vi "HFRR ADV v01.vi"() -> ()   [LabVIEW 2025] (continued)
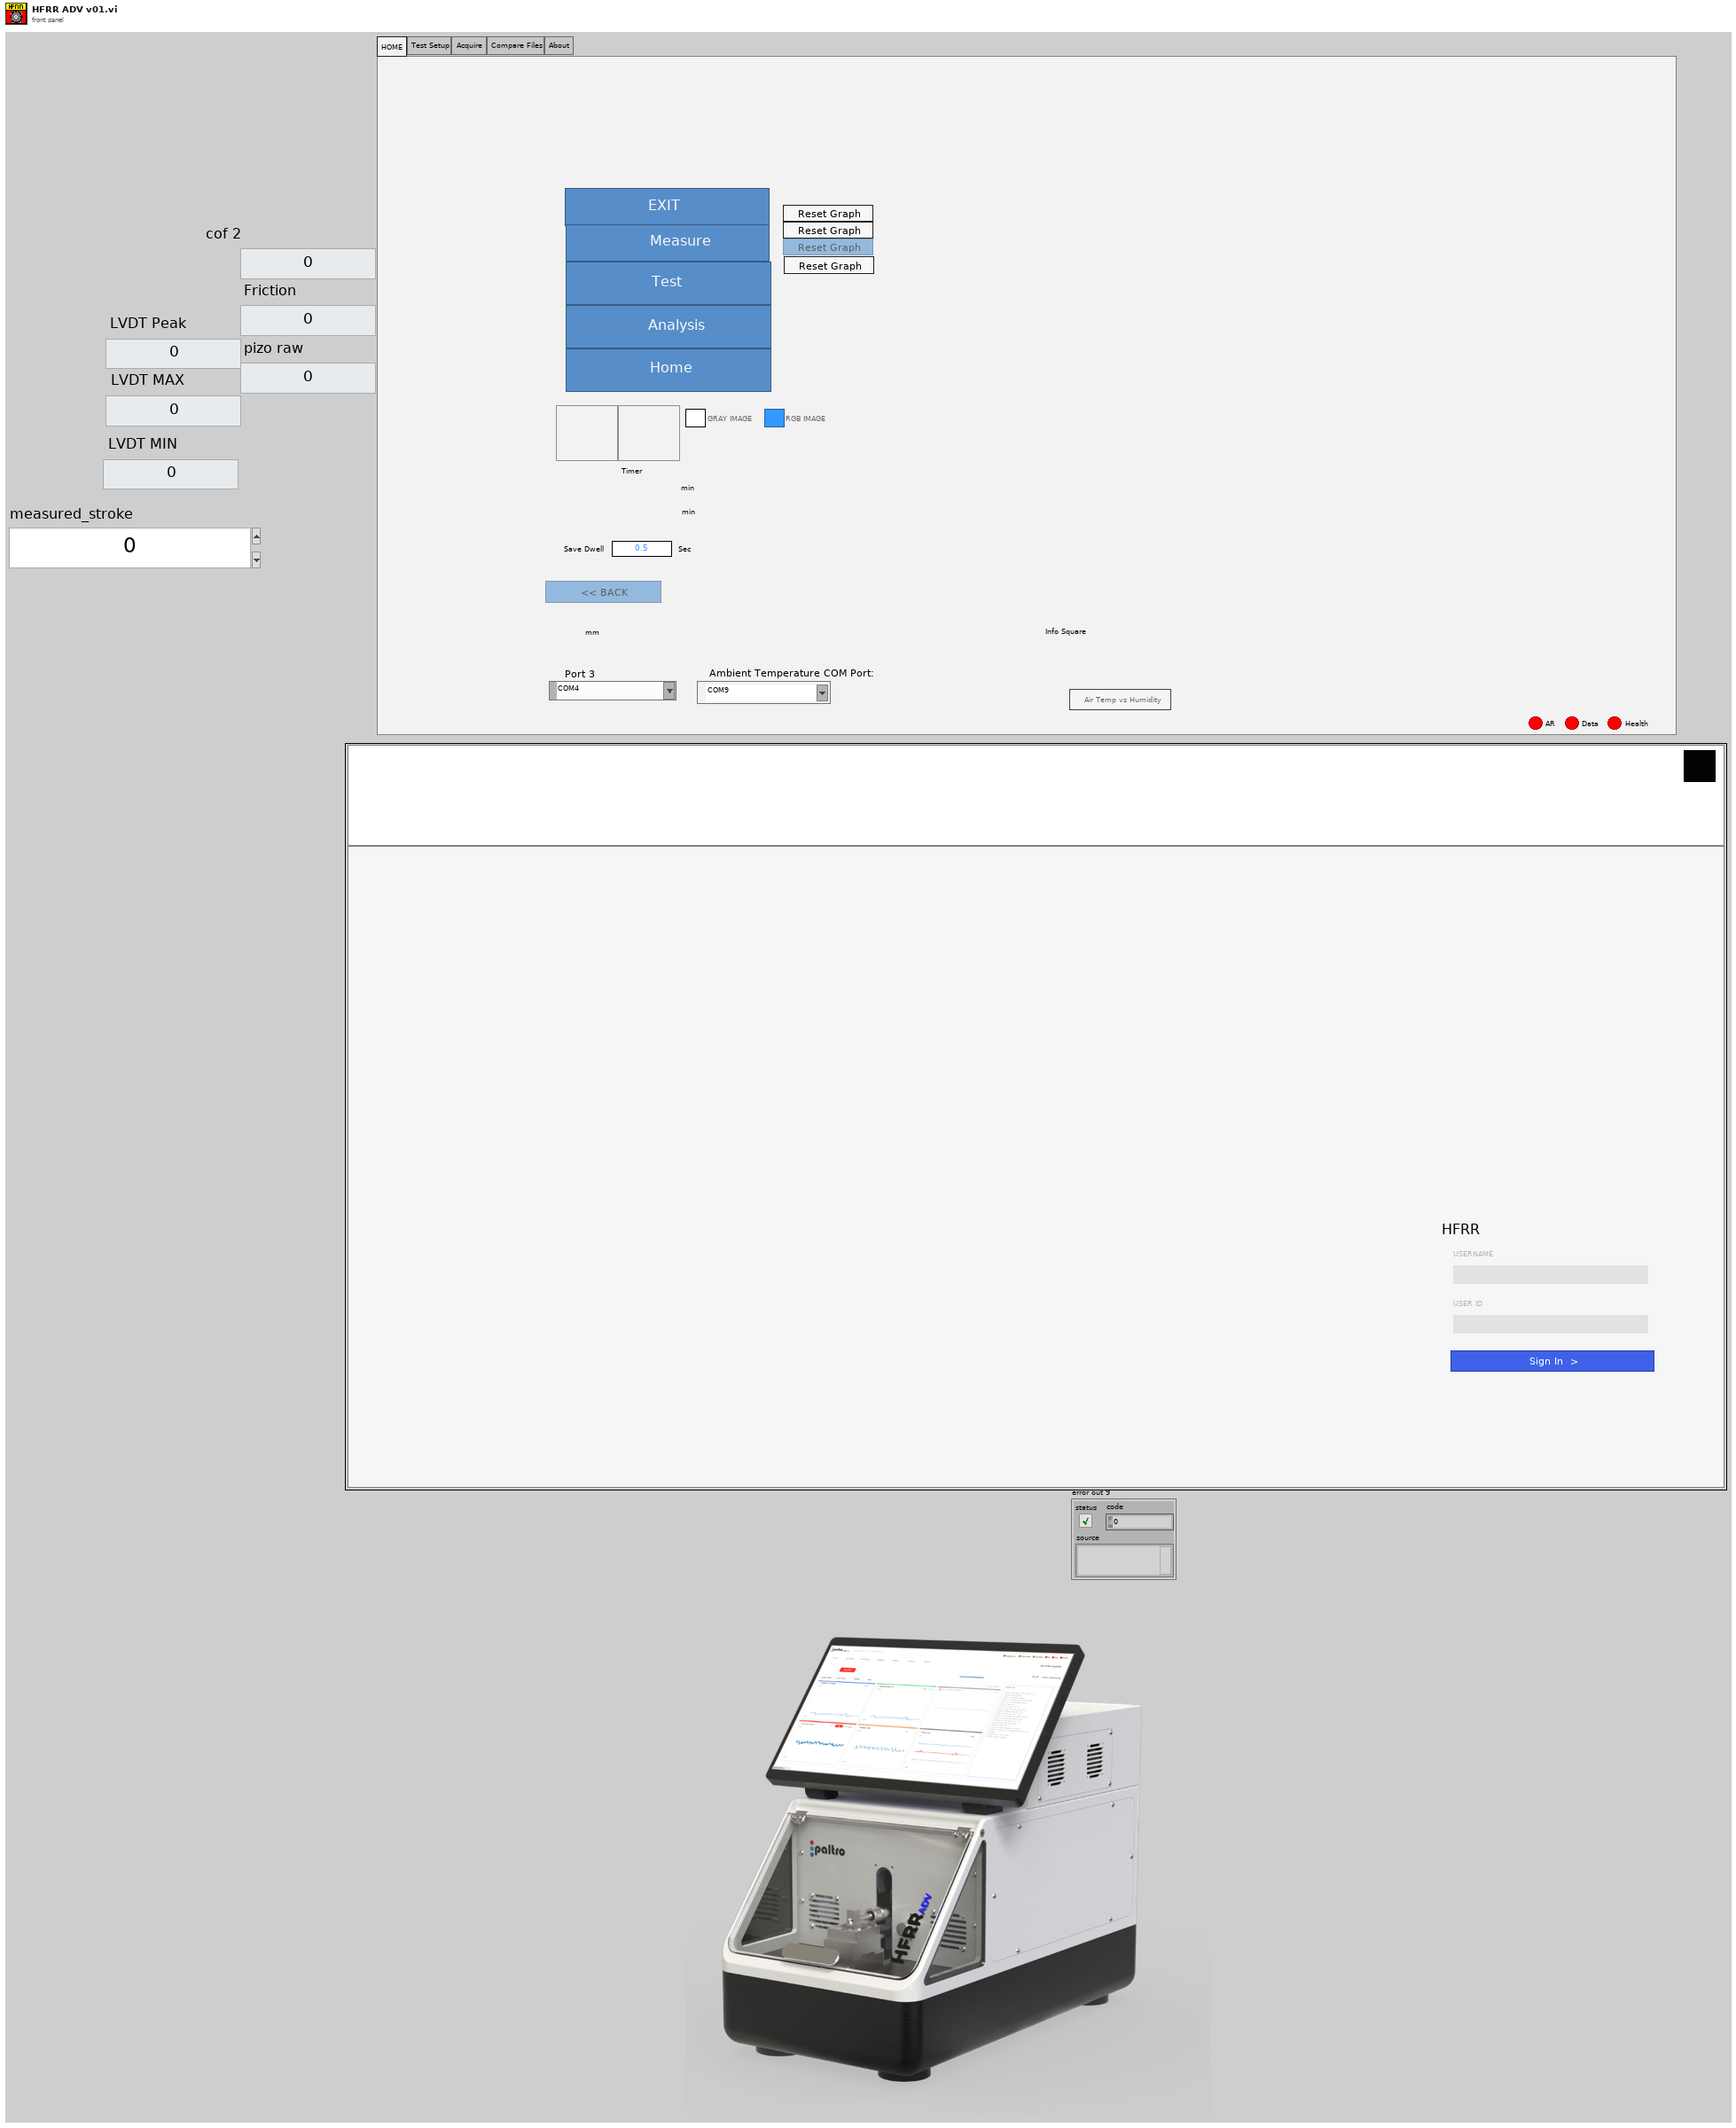
[diagram p1: front panel]
types:
  T1 = enum32{"Home", "Dashboard", "Imaging", "Report", "Analysis", "About", "Test Setup", "Advance"}
  T2 = enum32{"HOME", "Test Setup", "Acquire", "Adv Scar", "Adv Scar Report", "Compare Files", "About", "Advance", "Mooha"}
  T3 = enum16{"ASTM D6079", "ISO 12156", "CEC F-096-A-06", "Custom"}
  T4 = enum32{"Dashboard 1", "Dashboard 2", "Dashboard 3"}
  T5 = enum32{"COF", "Friction", "ECR", "Temperature", "Humidity", "Stroke"}
  T6 = enum32{"Coefficient Of Friction", "Air Temperature", "Humidity", "Stroke", "Sample Temperature", "Electrical Contact Resistance", "Frequency", "Air Temp vs Rh"}
  T7 = enum32{"Gains", "Configuration Parameters", "Temperature Calibration"}
  T8 = enum32{"Stroke Data", "Temperature Calibration", "Friction Force Raw Data"}
  T9 = enum32{"Temp Variables", "Camera", "WO 2465 (1)", "WO 2465 (2)", "WO 2465 (3)"}
  T10 = typedef "Auto Start enum.ctl" = enum16{"Init", "Humidity & Temperature On", "Reach point", "Maintain Stage", "Start Stage", "close", "Exit"}
  T11 = enum32{"Freqz control", "Low Speed Analog Inputs & Digital IOs", "Temperature Tuning", "Voltage LVDT raw", "High Speed Analog Inputs - Displacement & Friction", "LVDT Calibration", "Sericve", "Friction Force Calibration", "Bytes At Port", "Loadcell Board"}
  T12 = cluster{"proportional gain (Kc)":dbl, "integral time (Ti, min)":dbl, "derivative time (Td, min)":dbl}
  T13 = typedef "imagedata.ctl" = cluster{"image type":i32, "image depth":i32, "image":u8[], "mask":u8[], "colors":u32[], "Rectangle":cluster{"left":i16, "top":i16, "right":i16, "bottom":i16}}
  T14 = enum32{"HOME", "Test Setup", "Acquire", "Compare Files", "Print Report", "About", "Advance", "Mooha"}
  T15 = enum8{"Enabled", "Disabled", "Disabled and Grayed Out"}
  T16 = cluster{"Read Heave and Surge":string, "Bytes at Heave Port":dbl, "Heave and Surge COM Port:":refnum<visa-resource-name>, "Com Port 2":refnum<visa-resource-name>, "Residual Due":string, "Heave COM Status 2":bool, "Heave COM Status":bool, "Port 2":bool, "Sway PPR":dbl, "Surge PPR":dbl, "Heave PPR":dbl, "Sway Pitch":dbl, "Surge Pitch":dbl, "Heave Pitch":dbl, "Sway Pulses/mm":dbl, "Surge Pulses/mm":dbl, "Heave Pulses/mm":dbl, "inner loop":dbl, "Read Heave and Surge 2":string, "String 36":string, "Write S":bool, "WriteCC1":string[], "Heave COM Loop":i32, "LastCom":string, "EXIT":bool, "Error Heave":errorcluster}
  T17 = enum16{"Always On", "Always Off", "Off While Running"}
  T18 = typedef "POST ANALYSIS ENUM.ctl" = enum16{"OPEN EXE", "INIT", "OPEN FILE", "FIT", "DRAW REC", "DRAW LINE", "PAN", "ZOOM IN", "ZOOM OUT", "SET ZOOM", "CLEAR ROI", "GET MEASUREMENTS", "RESIZE MODE", "STREAM START", "STREAM STOP", "SHOW UI", "MINIMIZE UI", "HIDE UI", "CKISE APP", "CLOSE CONNECTION", "SAVE IMAGE", "SET ROI COLOR", "READ", "TCP CHECK", "CLOSE"}
  T19 = typedef "CAMERA LIVE FEED ENUM.ctl" = enum16{"OPEN EXE", "INIT", "READ", "CAMERA CONNECT", "CAMERA START", "CAMERA STOP", "CAMERA GRAY", "CAMERA RGB", "CAMERA MINIMIZE", "CAMERA CLOSE", "CAMERA MODE LIST", "CAMERA MODE SET", "CAMERA RESTORE", "CAMERA SAVE", "CLOSE"}
  T20 = cluster{"File Name":string, "Test Method":string, "Operator":string, "Fuel Description":string, "Date and time":string}
  T21 = enum32{"Home", "Dashboard", "Imaging", "Report", "Analysis", "About", "Test Setup"}
  T22 = enum32{"HOME", "Test Setup", "Acquire", "Compare Files", "About", "Advance", "Mooha"}
  T23 = enum16{"deny read/write", "deny write-only", "deny none"}
  T24 = typedef "NI_ReportGenerationCore.lvlib/HTML Report Image Alignment.ctl" = enum16{"(default)", "LEFT", "RIGHT", "TOP", "TEXTTOP", "MIDDLE", "ABSMIDDLE", "BASELINE", "BOTTOM", "ABSBOTTOM"}
  T25 = enum16{"open", "replace", "create", "open or create", "replace or create", "replace or create with confirmation"}
  T26 = enum16{"INIT", "READ", "MANUAL WRITE", "WRITE", "CLOSE", "ERROR INIT"}
  T27 = enum16{"open", "open or create", "create or replace", "create", "open (read only)"}
  T28 = cluster{"Mode":enum16{"RTU", "ASCII"}, "Slave Address":u8}
diagram:
  w5 = FALSE ("Visible")
  w6 = T15."Enabled" ("Disabled")
  w9 = FALSE ("Visible")
  w8 = FALSE ("Humidity Off Command")
  w28 = "" ("USER ID")
  (unwired) ""
  # "[CH1]    - FF\n[CH2]   - TEMPERATURE\n[CH3]    - Humidity\n[CH4]    - AIR TEMP\n[CH5]\\- Visa Uno\n[CH6] \\- Visa Due\n[CH7]  \\- file path\n[CH8]   - Displacement Gain\n[CHA]   - Stroke Gain\n[CHB]   - Stroke PID Gain\n[CHC]   -Language Selection\n[CHD]   -Power +\n[CHE]   -Power_\n[CHF]   -Heater\n[CHG]   -Humidity Wet\n[CHH]   -Humidity Dry\n[CHI]   -Integral Time \n[CHIJ   -Air intercept\n[CHI]   -Temp Intercept"
  n1 = flat-sequence {
    tunnel: [w78] -> w19
    tunnel: w19 -> [w92]
    tunnel: [w91] -> w18
    tunnel: ["ao0"] -> w21
    tunnel: w18 -> [_]
    tunnel: w21 -> [w157]
    tunnel: [w157] -> w20
    tunnel: w20 -> [w203]
    tunnel: [w201] -> w32
    tunnel: [w203] -> w31
    tunnel: w32 -> [w254]
    tunnel: w31 -> [w210]
    tunnel: [w254] -> w17
    tunnel: [w216] -> w16
    tunnel: [w204] -> w15
    tunnel: [w261] -> _
    tunnel: [w260] -> _
    tunnel: [w262] -> w55
    tunnel: w17 -> [w262]
    tunnel: w16 -> [w260]
    tunnel: w15 -> [w261]
    frame #0 {
      n2 = control-ref of="This VI"() -> (w66:refnum<vi>)
      n3 = property class="VI"(reference=w66) -> (reference out=w57:refnum<vi>, error out=w61:errorcluster, "Panel"=w65:refnum<vi>)  [unwired: 1 in]
      n4 = property class="Pnl"(reference=w65, error in=w61) -> (reference out=w59:refnum<vi>, error out=w62:errorcluster, "Panes[]"=w64:refnum<vi>[])
      n5 = for {
        tunnel: w64 -> [w72] mode=indexing
        tunnel: T17."Always Off" ("Horizontal Scrollbar Visibility") -> [w71]
        tunnel: w62 -> [w68]
        tunnel: [w67] -> w60
        n6 = property class="Pane"(reference=w72, error in=w68, "HorizScrollbarVisibility"=w71) -> (reference out=w69:refnum<vi>, error out=w70:errorcluster)
        n7 = Close Reference(reference=w69, error in (no error)=w70) -> (error out=w67:errorcluster)
      }
      n8 = Close Reference(reference=w59, error in (no error)=w60) -> (error out=w58:errorcluster)
      n9 = Close Reference(reference=w57, error in (no error)=w58) -> (error out=→"error out 8":errorcluster)
    }
    frame #1 {
      n10 = call "CLOSE CONNECTION.vi"("error in (no error)"="error in (no error) 2") -> ("error out"=w76:errorcluster)  [unwired: 10 in]
      n11 = call <vilib>:"Clear Errors.vi"("error in (no error)"=w76) -> ("error out"=w75:errorcluster)  [unwired: 5 in, 1 out]
      n12 = disable-structure shown="Enabled" {
        disable-tunnel: w75 -> [w82 _]
        disable-tunnel: [w81 _] -> w78
        frame Enabled {
          n13 = call <userlib>:"Fit VI window to Largest Dec.vi"("error in (no error)"=w82, "border spacing (2 px)"=1) -> ("error out"=w85:errorcluster, "dup VI Ref"=w89:refnum<vi>)  [unwired: 4 in]
          n14 = invoke on="Invoke Node" class="VI" method="FP.Run-Time Position.Maximized"(reference=w89, error in=w85) -> (error out=w86:errorcluster)  [unwired: 2 in, 3 out]
          n15 = call <vilib>:"Clear Errors.vi"("error in (no error)"=w86) -> ("error out"=w88:errorcluster)  [unwired: 5 in, 1 out]
          n16 = control-ref of="This VI"() -> (w80:refnum<vi>)
          n17 = invoke on="Invoke Node" class="VI" method="Default Vals.Reinit All"(reference=w80, error in=w88) -> (reference out=w84:refnum<vi>, error out=w83:errorcluster)  [unwired: 1 in, 1 out]
          n18 = Close Reference(reference=w84, error in (no error)=w83) -> (error out=w81:errorcluster)
        }
        frame Disabled {
        }
      }
      n19 = local write "sign in temp"(FALSE ("sign in temp")) -> ()
      n20 = property on="Sign In" class="Bool (strict)"("DisabledEnum"=T15."Disabled" ("Disabled")) -> ()  [unwired: 2 in, 2 out]
      n21 = property on="Auto Scar Check" class="Clust (strict)"("Visible"=TRUE) -> ()  [unwired: 2 in, 2 out]
    }
    frame #2 {
      n22 = call "dialog box.vi"("Status"="Before starting the test, verify that the microscope cable is connected.", "error in"=w92) -> ("error out"=w91:errorcluster)  [unwired: 8 in]
    }
    frame #3 {
      w99 = FALSE ("Upld AR 2")
      # "kkkkk"
      # "C:\\Windows\\wndcm_pw_stdED hfrr.txt"
      # "C:\\LAB-IQ NXT"
      # "C:\\LAB-IQ NXT\\wndcm_pw_stdED hfrr.txt"
      # "password file"
      n23 = Current VI's Path() -> (path=w112:path)
      n24 = Strip Path(path=w112) -> (stripped path=w105:path)  [unwired: 1 out]
      n25 = Path To String(path=w105) -> (string=w107:string)
      n26 = local write "conststatus"(0.0 ("rpm value : 2")) -> ()
      n27 = local write "Upld AR 2"(TRUE ("Upld AR 2")) -> ()
      n28 = local write "Lan flag"(0.0 ("Lan flag")) -> ()
      n29 = local write "COUNT"(0 ("COUNT")) -> ()
      n30 = local write "FLAG 2"(0.0 ("FLAG 2")) -> ()
      n31 = local write "Com flag"(u32 0 ("Com flag")) -> ()
      n32 = local write "Re-Initialise"(TRUE ("Re-Initialise")) -> ()
      n33 = local write "refresh flag"(FALSE ("refresh flag")) -> ()
      n34 = local write "Json St Flg"(w99) -> ()
      n35 = Search/Split String(string=w107, search string/char (-)=".exe") -> (match + rest of string=w109:string)  [unwired: 1 in, 2 out]
      n36 = Match True/False String(2:".vi" ("false string"), 3:".exe" ("true string"), 4:w109) -> (0:w106:bool)  [unwired: 1 out]
      n37 = local write "Json End Flg"(w99) -> ()
      n38 = case shown="True" w106 {
        tunnel: w105 -> [w128 w130]
        tunnel: [w128 w129] -> w103
        frame False {
        }
        frame True {
          n39 = Strip Path(path=w130) -> (stripped path=w129:path)  [unwired: 1 out]
        }
      }
      n40 = Path To String(path=w103) -> (string=→"Gain path":string)
      n41 = local write "Main Tab Display"(T4."Dashboard 1" ("Main Tab Display")) -> ()
      n42 = local write "main tab sub"(enum32{"Page 1", "Page 2"}."Page 1" ("main tab sub")) -> ()
      n43 = local write "Main Tab"(T2."HOME" ("Main Tab")) -> ()
      n44 = local write "EVENT LOG"("") -> ()
      n45 = List Folder(path=path "C:/LAB-IQ" ("directory path"), pattern="*.txt") -> (filenames=w118:string[])  [unwired: 2 in, 3 out]
      n46 = Search 1D Array(1D array=w118, element="wndcm_pw_stdED hfrr.txt") -> (index of element=w121:i32)  [unwired: 1 in]
      n47 = Equal?(x=w121, y=-1) -> (x = y?=w116:bool)
      n48 = case shown="True" w116 {
        frame False {
        }
        frame True {
          n49 = String To Byte Array(string="123\n") -> (unsigned byte array=w135:u8[])
          n50 = Array Size(array=w135) -> (size(s)=w134:i32)
          n51 = for {
            N: w134 -> [_]
            tunnel: w135 -> [w148]
            tunnel: [w145] -> w137 mode=indexing
            tunnel: w134 -> [w140]
            i -> [w138]
            n52 = Decrement(x=w140) -> (x-1=w141:i32)
            n53 = Equal?(x=w138, y=w141) -> (x = y?=w142:bool)
            n54 = Index Array(array=w148, index=w138) -> (element=w147:u8)
            n55 = Number To Decimal String(number=w147) -> (decimal integer string=w146:string)  [unwired: 1 in]
            n56 = Select(t="", s=w142, f="\r") -> (s? t:f=w139:string)
            n57 = Concatenate Strings(w146, w139) -> (w145:string)
          }
          n58 = local read "file path"() -> (w131:path)
          n59 = Concatenate Strings(w137) -> (w133:string)
          n60 = call <vilib>:"Write Characters To File.vi"("append to file? (new file:F)"=FALSE, "character string"=w133, "file path (dialog if empty)"=w131) -> ()  [unwired: 2 in, 1 out]
        }
      }
      n61 = local write "clk"(0.0 ("clk")) -> ()
      n62 = local write "Flag"(0.0 ("Flag")) -> ()
      "file path" <- path "C:/LAB-IQ/wndcm_pw_stdED hfrr.txt" ("file path")
      "FF buffer" <- dbl[] [] ("FF buffer")
    }
    frame #4 {
      # "C:\\WinDucom\\calibrate WO 2391.dcf"
      n63 = String To Path(string="C:\\LAB-IQ\\calibrate WO 2465.dcf") -> (path=w156:path)
      n64 = Open/Create/Replace File "Open File"(file path (use dialog)=w156) -> (refnum out=w155:refnum<file>)  [unwired: 5 in, 2 out]
      n65 = for {
        N: 24 -> [_]
        tunnel: w155 -> [w176]
        i -> [w170]
        (unwired) TRUE ("line mode (F)")
        n66 = Read from Text File "Read File"(file (use dialog)=w176) -> (text=w175:string)  [unwired: 3 in, 3 out]
        n67 = Match Pattern(string=w175, regular expression="]") -> (after substring=w173:string)  [unwired: 1 in, 3 out]
        n68 = String Subset(string=w175, offset (0)=5, length (rest)=10 ("length (rest)")) -> (substring=w168:string)
        n69 = Fract/Exp String To Number(string=w168) -> (number=w169:dbl)  [unwired: 3 in, 1 out]
        n70 = Match Pattern(string=w173, regular expression="-") -> (before substring=w171:string)  [unwired: 1 in, 3 out]
        n71 = case shown="20" w170 {
          tunnel: w169 -> [w179 w180 w181 w182 _ _ _ w187 w188 _ w189 w190 w191 w192 w193 w194 _ w195 w196 _ _ _ _ _ _]
          tunnel: w171 -> [_ _ _ _ w183 w184 w185 _ _ _ _ _ _ _ _ _ _ _ _ w197 w198 _ w199 w200 _]
          frame 0 {
            n72 = local write "FRIC. FORCE :"(w179) -> ()
          }
          frame 1 {
            n73 = local write "TEMPERATURE :"(w180) -> ()
          }
          frame 2 {
            n74 = local write "HUMIDITY:"(w181) -> ()
          }
          frame 3 {
            n75 = local write "AIR TEMPERATURE :"(w182) -> ()
          }
          frame 4 {
            n76 = local write "Com Port 1"(w183) -> ()
          }
          frame 5 {
            n77 = local write "Com Port 2"(w184) -> ()
            n78 = local write "visa due"(w184) -> ()
          }
          frame 6 {
            n79 = String To Path(string=w185) -> (path=w186:path)
            n80 = local write "File Path"(w186) -> ()
          }
          frame 7 {
            n81 = local write "DISPLACEMENT :"(w187) -> ()
          }
          frame 8 {
            n82 = local write "STROKE GAIN :"(w188) -> ()
          }
          frame 9 {
          }
          frame 10 {
            n83 = local write "Language Selection"(w189) -> ()
          }
          frame 11 {
            n84 = local write "CH-POWER +"(w190) -> ()
          }
          frame 12 {
            n85 = local write "CH-POWER -"(w191) -> ()
          }
          frame 13 {
            n86 = local write "CH-HEATER"(w192) -> ()
          }
          frame 14 {
            n87 = local write "CH-HUMIDITY WET"(w193) -> ()
          }
          frame 15 {
            n88 = local write "CH-HUMIDITY DRY"(w194) -> ()
          }
          frame 16 {
          }
          frame 17 {
            n89 = local write "AIR TEMP INTERCEPT:"(w195) -> ()
          }
          frame 18 {
            n90 = local write "TEMP INTERCEPT:"(w196) -> ()
          }
          frame 19 {
            n91 = local write "S.NO"(w197) -> ()
          }
          frame 20 {
            n92 = local write "Com Port 3"(w198) -> ()
          }
          frame 21 {
          }
          frame 22 {
            n93 = local write "C3 :"(w199) -> ()
          }
          frame 23 {
            n94 = local write "Camera Port :"(w200) -> ()
          }
          frame 24, Default {
          }
        }
      }
      n95 = String To Path(string="C:\\LAB-IQ\\Image Calibrate v01.dcf") -> (path=w152:path)
      n96 = Open/Create/Replace File ("Open File")(file path (use dialog)=w152) -> (refnum out=w151:refnum<file>)  [unwired: 5 in, 2 out]
      n97 = for {
        N: 4 -> [_]
        tunnel: w151 -> [w163]
        i -> [w159]
        n98 = Read from Text File ("Read File")(file (use dialog)=w163) -> (text=w164:string)  [unwired: 3 in, 3 out]
        n99 = String Subset(string=w164, offset (0)=6, length (rest)=10 ("length (rest)")) -> (substring=w160:string)
        n100 = Fract/Exp String To Number(string=w160) -> (number=w158:dbl)  [unwired: 3 in, 1 out]
        n101 = case shown="3" w159 {
          tunnel: w158 -> [w165 w166 _ w167 _]
          frame 0 {
            n102 = local write "5x Gain"(w165) -> ()
          }
          frame 1 {
            n103 = local write "10x Gain"(w166) -> ()
          }
          frame 2 {
          }
          frame 3 {
            n104 = local write "100x gain"(w167) -> ()
          }
          frame 4, Default {
          }
        }
      }
    }
    frame #5 {
      n105 = Wait (ms)(milliseconds to wait=u32 1000) -> (millisecond timer value=w201:u32)
    }
    frame #6 {
      w219 = u32 2000 ("milliseconds to wait")
      w246 = u32 2000 ("milliseconds to wait")
      n106 = local read "Re-Initialise"() -> (w253:bool)
      n107 = case shown="True" w253 {
        frame False {
        }
        frame True {
          n108 = local write "Re-Initialise"(FALSE ("Re-Initialise")) -> ()
        }
      }
      n109 = call "CAMERA LIVE FEED FGV.vi"("Enum - Menu"=CAMERA_LIVE_FEED_ENUM."OPEN EXE", "error in (no error)"=w210) -> ("error out"=w252:errorcluster)  [unwired: 8 in, 1 out]
      n110 = call "Stall Data Flow.vim"("value in"=w252, "milliseconds to wait"=w246) -> ("value out"=w250:errorcluster)  [unwired: 1 out]
      n111 = call "CAMERA LIVE FEED FGV.vi"("Enum - Menu"=CAMERA_LIVE_FEED_ENUM."INIT", "error in (no error)"=w250) -> ("error out"=w248:errorcluster)  [unwired: 8 in, 1 out]
      n112 = call "IMAGE ANALYSIS.vi"("Enum"=POST_ANALYSIS_ENUM."OPEN EXE", "error in"=w210) -> ("error out"=w207:errorcluster)  [unwired: 8 in, 1 out]
      n113 = case shown="Error .." w248 {
        selector: w248 -> [w255 _]
        tunnel: [w255 _] -> w247
        frame No Error {
        }
        frame Error {
          n114 = One Button Dialog(message="Camera initialization error.\nPlease Restart the software") -> ()  [unwired: 1 in, 1 out]
        }
      }
      n115 = call "Stall Data Flow.vim"("value in"=w207, "milliseconds to wait"=u32 8000) -> ("value out"=w206:errorcluster)  [unwired: 1 out]
      n116 = property on="Camera Port :" class="CmbBox"() -> ("Strings[]"=w244:string[], "Value"=w245:string)  [unwired: 2 in, 2 out]
      n117 = call "IMAGE ANALYSIS.vi"("Enum"=POST_ANALYSIS_ENUM."INIT", "error in"=w206) -> ("error out"=w204:errorcluster)  [unwired: 8 in, 1 out]
      n118 = Search 1D Array(1D array=w244, element=w245) -> (index of element=w243:i32)  [unwired: 1 in]
      n119 = Type Cast(type=30, x=w243) -> (*(type *) &x=w241:i32)
      n120 = call "Stall Data Flow.vim"("value in"=w247, "milliseconds to wait"=w246) -> ("value out"=w223:errorcluster)  [unwired: 1 out]
      n121 = Add(x=w241, y=48) -> (x+y=w222:i32)
      n122 = call "CAMERA LIVE FEED FGV.vi"("Enum - Menu"=CAMERA_LIVE_FEED_ENUM."CAMERA CONNECT", "error in (no error)"=w223, "CAMERA PORT"=w222) -> ("error out"=w232:errorcluster)  [unwired: 7 in, 1 out]
      n123 = call "Stall Data Flow.vim"("value in"=w232, "milliseconds to wait"=u32 5000) -> ("value out"=w233:errorcluster)  [unwired: 1 out]
      n124 = call "CAMERA LIVE FEED FGV.vi"("Enum - Menu"=CAMERA_LIVE_FEED_ENUM."CAMERA MODE LIST", "error in (no error)"=w233) -> ("error out"=w235:errorcluster)  [unwired: 8 in, 1 out]
      n125 = call "Stall Data Flow.vim"("value in"=w235, "milliseconds to wait"=w219) -> ("value out"=w234:errorcluster)  [unwired: 1 out]
      n126 = call "CAMERA LIVE FEED FGV.vi"("Enum - Menu"=CAMERA_LIVE_FEED_ENUM."READ", "error in (no error)"=w234) -> ("error out"=w221:errorcluster, "data out"=→"Camera List":string)  [unwired: 8 in]
      n127 = call "Stall Data Flow.vim"("value in"=w221, "milliseconds to wait"=w219) -> ("value out"=w220:errorcluster)  [unwired: 1 out]
      n128 = Type Cast(type=30, x=0) -> (*(type *) &x=w215:i32)
      n129 = Add(x=w215, y=48) -> (x+y=w213:i32)
      n130 = call "CAMERA LIVE FEED FGV.vi"("Enum - Menu"=CAMERA_LIVE_FEED_ENUM."CAMERA MODE SET", "error in (no error)"=w220, "CAMERA MODE"=w213) -> ("error out"=w217:errorcluster)  [unwired: 7 in, 1 out]
      n131 = call "Stall Data Flow.vim"("value in"=w217, "milliseconds to wait"=u32 2000) -> ("value out"=w237:errorcluster)  [unwired: 1 out]
      n132 = call "CAMERA LIVE FEED FGV.vi"("Enum - Menu"=CAMERA_LIVE_FEED_ENUM."CAMERA START", "error in (no error)"=w237) -> ("error out"=w238:errorcluster)  [unwired: 8 in, 1 out]
      n133 = call "Stall Data Flow.vim"("value in"=w238, "milliseconds to wait"=u32 1000) -> ("value out"=w239:errorcluster)  [unwired: 1 out]
      n134 = call "CAMERA LIVE FEED FGV.vi"("Enum - Menu"=CAMERA_LIVE_FEED_ENUM."CAMERA MINIMIZE", "error in (no error)"=w239) -> ("error out"=w216:errorcluster)  [unwired: 8 in, 1 out]
    }
    frame #7 {
      n135 = case shown="No Error" w260 {
        frame No Error {
          n136 = property on="Auto Scar Check" class="Clust (strict)"("Visible"=FALSE) -> ()  [unwired: 2 in, 2 out]
        }
        frame Error {
        }
      }
      n137 = local write "sign in temp"(TRUE ("sign in temp")) -> ()
      n138 = property on="Sign In" class="Bool (strict)"("DisabledEnum"=T15."Enabled" ("Disabled")) -> ()  [unwired: 2 in, 2 out]
    }
  }
  n139 = local write "Cal Password"("" ("Cal Password")) -> ()
  n140 = property on="Auto Start Test" class="Bool (strict)"("Visible"=TRUE) -> ()  [unwired: 2 in, 2 out]
  n141 = property on="FRICVALZ 2" class="Bool (strict)"("DisabledEnum"=w6) -> ()  [unwired: 2 in, 2 out]
  n142 = property on="FRICVALZ 4" class="Bool (strict)"("DisabledEnum"=w6) -> ()  [unwired: 2 in, 2 out]
  n143 = property on="FRICVALZ 3" class="Bool (strict)"("DisabledEnum"=w6) -> ()  [unwired: 2 in, 2 out]
  n144 = property on="About" class="Clust (strict)"("Visible"=FALSE) -> ()  [unwired: 2 in, 2 out]
  n145 = property on="Tab Control 5" class="TabCtl (strict)"("Tabs Visible?"=TRUE ("Page Labels Display Visible?")) -> ()  [unwired: 2 in, 2 out]
  n146 = property on="Wrong Password" class="Str"("Visible"=w5) -> ()  [unwired: 2 in, 2 out]
  n147 = property on="Calibration 2" class="TabCtl (strict)"("Visible"=w5) -> ()  [unwired: 2 in, 2 out]
  n148 = local write "SCAR MEASURMENT"(enum32{"Auto Scar", "Manual Scar"}."Manual Scar" ("SCAR MEASURMENT")) -> ()
  n149 = local write "Temperature Off Command"(w8) -> ()
  n150 = local write "Main Dashboard Buttons"(T1."Home" ("Main Dashboard Buttons")) -> ()
  n151 = local write "Humidity Off Command"(w8) -> ()
  n152 = local write "CAMERA ROI MIN TEMP"(w8) -> ()
  n153 = local write "TEST FILE NAM,E SAVED"(w8) -> ()
  n154 = local write "LIVE FEED MIN TEMP"(w8) -> ()
  n155 = local write "SCAR MEASURMENT"(enum32{"Auto Scar", "Manual Scar"}."Manual Scar" ("SCAR MEASURMENT")) -> ()
  n156 = while {
    stop <- w264 stop-if-true
    n157 = event shown="[1] \"RUN\": Value Change" {
      selector: _ -> [_ _ _ _ _ _ _ _ _ _ _ _ _]
      dyn-events: _ -> [_ _ _ _ _ _ _ _ _ _ _ _ _]
      timeout: 100 -> [_ _ _ _ _ _ _ _ _ _ _ _ _]
      tunnel: [FALSE FALSE _ FALSE _ _ _ _ _ _ _ _ TRUE] -> w264
      event Timeout {
        n158 = event-data() -> ()  [unwired: 1 in, 3 out]
        n159 = local read "Auto Start Test"() -> (w268:bool)
        n160 = local read "RUN"() -> (w269:bool)
        n161 = Or(x=w269, y=w268) -> (x .or. y?=w267:bool)
        n162 = case shown="True" w267 {
          frame False {
            w280 = TRUE ("PAUSE")
            n163 = call "ELAPSED TIMER VI - abort test.vi"("RESET"=w280, "PAUSE"=w280) -> ()  [unwired: 7 in, 3 out]
          }
          frame True {
            n164 = local read "Stroke 2"() -> (w285:dbl)
            n165 = local read "FF 3"() -> (w287:dbl)
            n166 = Equal?(x=w285, y=0.95 ("Stroke 2")) -> (x = y?=w282:bool)
            n167 = Equal?(x=w287, y=0.0 ("FF 3")) -> (x = y?=w283:bool)
            n168 = Or(x=w283, y=w282) -> (x .or. y?=w281:bool)
            n169 = case shown="True" w281 {
              selector: w281 -> [_ w292]
              frame False {
                w288 = TRUE ("PAUSE")
                n170 = call "ELAPSED TIMER VI - abort test.vi"("RESET"=w288, "PAUSE"=w288) -> ()  [unwired: 7 in, 3 out]
              }
              frame True {
                n171 = Not(x=w292) -> (.not. x?=w291:bool)
                n172 = call "ELAPSED TIMER VI - abort test.vi"("TARGET"=60.0, "RESET"=w291, "PAUSE"=FALSE) -> ("ELAPSED INDICATION"=w289:bool)  [unwired: 6 in, 2 out]
                n173 = case shown="True" w289 {
                  frame False {
                  }
                  frame True {
                    n174 = stacked-sequence {
                      frame #0 {
                        w294 = FALSE
                        n175 = local write "RUN"(w294) -> ()
                        n176 = local write "Auto Start Test"(w294) -> ()
                      }
                      frame #1 {
                        n177 = One Button Dialog(message="Test stopped due to a communication error. Reconnect the C1 and C2 cables.") -> ()  [unwired: 1 in, 1 out]
                      }
                    }
                  }
                }
              }
            }
          }
        }
        n178 = Get Date/Time In Seconds() -> (seconds since 1Jan1904=w278:timestamp)
        n179 = Format Into String(format string="%<%I:%M:%S:%p %d:%B:%Y>T", w278) -> (resulting string=→"Time Stamp":string)  [unwired: 2 in, 1 out]
        n180 = local read "Service Password enable"() -> (w270:bool)
        n181 = local read "FILE"() -> (w275:string)
        n182 = call <vilib>:"Trim Whitespace.vi"("string"=w275) -> ("trimmed string"=w274:string)  [unwired: 1 in]
        n183 = String Length(string=w274) -> (length=w273:i32)
        n184 = Greater?(x=w273, y=1) -> (0:w271:bool)
        n185 = case shown="False" w271 {
          tunnel: w270 -> [w296 _]
          frame False {
            n186 = case shown="True" w296 {
              frame True {
                w297 = "Test Start In Service Mode" ("Tip Strip")
                w298 = T15."Enabled" ("Disabled")
                n187 = property on="Auto Start Test" class="Bool (strict)"("DisabledEnum"=w298, "TipStrip"=w297) -> ()  [unwired: 2 in, 2 out]
                n188 = property on="RUN" class="Bool (strict)"("DisabledEnum"=w298, "TipStrip"=w297) -> ()  [unwired: 2 in, 2 out]
              }
              frame False {
                w299 = "Enter File Name to Start Test" ("Tip Strip")
                w300 = T15."Disabled and Grayed Out" ("Disabled")
                n189 = property on="Auto Start Test" class="Bool (strict)"("DisabledEnum"=w300, "TipStrip"=w299) -> ()  [unwired: 2 in, 2 out]
                n190 = property on="RUN" class="Bool (strict)"("DisabledEnum"=w300, "TipStrip"=w299) -> ()  [unwired: 2 in, 2 out]
              }
            }
          }
          frame True {
            w301 = "" ("Tip Strip")
            w302 = T15."Enabled" ("Disabled")
            n191 = property on="Auto Start Test" class="Bool (strict)"("DisabledEnum"=w302, "TipStrip"=w301) -> ()  [unwired: 2 in, 2 out]
            n192 = property on="RUN" class="Bool (strict)"("DisabledEnum"=w302, "TipStrip"=w301) -> ()  [unwired: 2 in, 2 out]
          }
        }
      }
      event "RUN": Value Change {
        n193 = event-data() -> ()  [unwired: 1 in, 6 out]
        n194 = local read "RUN"() -> (w304:bool)
        n195 = case shown="True" w304 {
          frame False {
            w305 = T15."Enabled" ("Disabled")
            w309 = "" ("FILE")
            n196 = local write "FILE"(w309) -> ()
            n197 = local write "Batch Ref Num :"(w309) -> ()
            n198 = local write "Fuel Discription :"(w309) -> ()
            n199 = local write "Main Tab"(T2."Adv Scar" ("Main Tab")) -> ()
            n200 = local write "Remarks :"(w309) -> ()
            n201 = local write "Main Dashboard Buttons"(T1."Imaging" ("Main Dashboard Buttons")) -> ()
            n202 = local write "TEST FILE NAM,E SAVED"(FALSE ("TEST FILE NAM,E SAVED")) -> ()
            n203 = property on="Stroke ( mm )" class="WFChart (strict)"("History Data"=cluster{"y":dbl, dbl, "y":dbl}[] []) -> ()  [unwired: 2 in, 2 out]
            n204 = property on="Auto Start Test" class="Bool (strict)"("Visible"=TRUE) -> ()  [unwired: 2 in, 2 out]
            n205 = property on="FRICVALZ 2" class="Bool (strict)"("DisabledEnum"=w305) -> ()  [unwired: 2 in, 2 out]
            n206 = property on="FRICVALZ 4" class="Bool (strict)"("DisabledEnum"=w305) -> ()  [unwired: 2 in, 2 out]
            n207 = property on="FRICVALZ 3" class="Bool (strict)"("DisabledEnum"=w305) -> ()  [unwired: 2 in, 2 out]
          }
          frame True {
            w312 = T15."Disabled" ("Disabled")
            n208 = property on="Auto Start Test" class="Bool (strict)"("Visible"=FALSE) -> ()  [unwired: 2 in, 2 out]
            n209 = property on="FRICVALZ 2" class="Bool (strict)"("DisabledEnum"=w312) -> ()  [unwired: 2 in, 2 out]
            n210 = property on="FRICVALZ 4" class="Bool (strict)"("DisabledEnum"=w312) -> ()  [unwired: 2 in, 2 out]
            n211 = property on="FRICVALZ 3" class="Bool (strict)"("DisabledEnum"=w312) -> ()  [unwired: 2 in, 2 out]
          }
        }
      }
      event "Auto": Value Change {
        n212 = event-data() -> ()  [unwired: 1 in, 6 out]
        n213 = stacked-sequence {
          frame #0 {
            n214 = local write "FILE"("") -> ()
          }
          frame #1 {
            n215 = Get Date/Time In Seconds() -> (seconds since 1Jan1904=w318:timestamp)
            n216 = Format Into String(format string="%<%I_%M_%S_%p_%d_%B_%Y>T", w318) -> (resulting string=w317:string)  [unwired: 2 in, 1 out]
            n217 = local write "FILE"(w317) -> ()
          }
        }
        n218 = local read "Auto"() -> (w315:bool)
        n219 = Not(x=w315) -> (.not. x?=w314:bool)
        n220 = local write "Auto"(w314) -> ()
      }
      event "Auto Start Test": Value Change {
        n221 = event-data() -> ()  [unwired: 1 in, 6 out]
        n222 = local read "Auto Start Test"() -> (w321:bool)
        n223 = case shown="True" w321 {
          frame False {
            w322 = T15."Enabled" ("Disabled")
            w326 = "" ("FILE")
            n224 = local write "Main Tab"(T2."Adv Scar" ("Main Tab")) -> ()
            n225 = local write "Main Dashboard Buttons"(T1."Imaging" ("Main Dashboard Buttons")) -> ()
            n226 = property on="RUN" class="Bool (strict)"("Visible"=TRUE) -> ()  [unwired: 2 in, 2 out]
            n227 = local write "TEST FILE NAM,E SAVED"(FALSE ("TEST FILE NAM,E SAVED")) -> ()
            n228 = local write "Fuel Discription :"(w326) -> ()
            n229 = local write "Batch Ref Num :"(w326) -> ()
            n230 = local write "Remarks :"(w326) -> ()
            n231 = local write "FILE"(w326) -> ()
            n232 = property on="FRICVALZ 2" class="Bool (strict)"("DisabledEnum"=w322) -> ()  [unwired: 2 in, 2 out]
            n233 = property on="FRICVALZ 4" class="Bool (strict)"("DisabledEnum"=w322) -> ()  [unwired: 2 in, 2 out]
            n234 = property on="FRICVALZ 3" class="Bool (strict)"("DisabledEnum"=w322) -> ()  [unwired: 2 in, 2 out]
          }
          frame True {
            w328 = T15."Disabled" ("Disabled")
            n235 = property on="RUN" class="Bool (strict)"("Visible"=FALSE) -> ()  [unwired: 2 in, 2 out]
            n236 = property on="FRICVALZ 2" class="Bool (strict)"("DisabledEnum"=w328) -> ()  [unwired: 2 in, 2 out]
            n237 = property on="FRICVALZ 4" class="Bool (strict)"("DisabledEnum"=w328) -> ()  [unwired: 2 in, 2 out]
            n238 = property on="FRICVALZ 3" class="Bool (strict)"("DisabledEnum"=w328) -> ()  [unwired: 2 in, 2 out]
          }
        }
      }
      event "FILE", "USERNAME", "USER ID": Mouse Enter {
        n239 = event-data() -> ()  [unwired: 1 in, 4 out]
        n240 = dll-call lib="kernel32.dll" fn="Wow64DisableWow64FsRedirection"("OldValue"=0) -> (error out=w335:errorcluster, "OldValue"=w333:i32)  [unwired: 4 in, 1 out]
        n241 = call <vilib>:"System Exec.vi"("run minimized? (F)"=TRUE, "error in (no error)"=w335, "command line"="C:\\Program Files\\Common Files\\Microsoft Shared\\Ink\\TabTip.exe") -> ("error out"=w334:errorcluster)  [unwired: 5 in, 3 out]
        n242 = dll-call lib="kernel32.dll" fn="Wow64EnableWow64FsRedirection"(error in=w334, "OldValue"=w333) -> ()  [unwired: 4 in, 2 out]
      }
      event "EDIT": Value Change {
        n243 = event-data() -> ()  [unwired: 1 in, 6 out]
        n244 = local read "EDIT"() -> (w336:bool)
        n245 = case shown="False" w336 {
          frame False {
            n246 = control-ref of="This VI"() -> (w353:refnum<vi>)
            n247 = property class="VI"(reference=w353) -> (reference out=w344:refnum<vi>, error out=w348:errorcluster, "Panel"=w352:refnum<vi>)  [unwired: 1 in]
            n248 = property class="Pnl"(reference=w352, error in=w348) -> (reference out=w346:refnum<vi>, error out=w349:errorcluster, "Panes[]"=w351:refnum<vi>[])
            n249 = for {
              tunnel: w351 -> [w359] mode=indexing
              tunnel: T17."Always Off" ("Horizontal Scrollbar Visibility") -> [w358]
              tunnel: w349 -> [w355]
              tunnel: [w354] -> w347
              n250 = property class="Pane"(reference=w359, error in=w355, "HorizScrollbarVisibility"=w358) -> (reference out=w356:refnum<vi>, error out=w357:errorcluster)
              n251 = Close Reference(reference=w356, error in (no error)=w357) -> (error out=w354:errorcluster)
            }
            n252 = Close Reference(reference=w346, error in (no error)=w347) -> (error out=w345:errorcluster)
            n253 = Close Reference(reference=w344, error in (no error)=w345) -> (error out=w339:errorcluster)
            "error out 7" <- w339
            n254 = call <vilib>:"Clear Errors.vi"("error in (no error)"=w339) -> ("error out"=w338:errorcluster)  [unwired: 5 in, 1 out]
            n255 = local write "Service Password enable"(FALSE ("Service Password enable")) -> ()
            n256 = call <userlib>:"Fit VI window to Largest Dec.vi"("error in (no error)"=w338, "border spacing (2 px)"=1) -> ("error out"=w343:errorcluster, "dup VI Ref"=w341:refnum<vi>)  [unwired: 4 in]
            n257 = invoke on="Invoke Node" class="VI" method="FP.Run-Time Position.Maximized"(reference=w341, error in=w343) -> (error out=w342:errorcluster)  [unwired: 2 in, 3 out]
            n258 = call <vilib>:"Clear Errors.vi"("error in (no error)"=w342) -> ()  [unwired: 5 in, 2 out]
          }
          frame True {
          }
        }
      }
      event "Headen Service Button": Value Change {
        n259 = event-data() -> ()  [unwired: 1 in, 6 out]
        n260 = local read "Headen Service Button"() -> (w360:bool)
        n261 = case shown="True" w360 {
          frame False {
            n262 = property on="Password 3" class="Clust (strict)"("Visible"=FALSE) -> ()  [unwired: 2 in, 2 out]
            n263 = property on="Service Password Log" class="Str"("Visible"=FALSE) -> ()  [unwired: 2 in, 2 out]
          }
          frame True {
            n264 = property on="Password 3" class="Clust (strict)"("Visible"=TRUE) -> ()  [unwired: 2 in, 2 out]
            n265 = property on="Service Password Log" class="Str"("Visible"=TRUE) -> ()  [unwired: 2 in, 2 out]
          }
        }
      }
      event "Password 3.Service Password": Value Change {
        n266 = event-data() -> ()  [unwired: 1 in, 6 out]
        n267 = Unbundle By Name("Password 3") -> ("Service Password"=w367:string)
        n268 = call <vilib>:"Trim Whitespace.vi"("string"=w367) -> ("trimmed string"=w365:string)  [unwired: 1 in]
        n269 = Equal?(x=w365, y="Service@123") -> (x = y?=w366:bool)
        n270 = case shown="False" w366 {
          selector: w366 -> [w371 w373]
          frame False {
            n271 = local write "Service Password enable"(w371) -> ()
            n272 = property on="Service Password Log" class="Str"("Visible"=TRUE) -> ()  [unwired: 2 in, 2 out]
            n273 = property on="Tab Control 5" class="TabCtl (strict)"("Tabs Visible?"=TRUE ("Page Labels Display Visible?")) -> ()  [unwired: 2 in, 2 out]
          }
          frame True {
            n274 = property on="Service Password Log" class="Str"("Visible"=FALSE) -> ()  [unwired: 2 in, 2 out]
            "Service Password enable" <- w373
          }
        }
      }
      event "Sign In": Value Change {
        w375 = FALSE ("Visible")
        n275 = event-data() -> ()  [unwired: 1 in, 6 out]
        n276 = property on="About" class="Clust (strict)"("Visible"=w375) -> ()  [unwired: 2 in, 2 out]
        n277 = property on="Password 3" class="Clust (strict)"("Visible"=w375) -> ()  [unwired: 2 in, 2 out]
        n278 = property on="Service Password Log" class="Str"("Visible"=FALSE) -> ()  [unwired: 2 in, 2 out]
      }
      event "Info": Value Change {
        n279 = event-data() -> ()  [unwired: 1 in, 6 out]
        n280 = local read "Info"() -> (w377:bool)
        n281 = case shown="False" w377 {
          frame False {
            n282 = property on="About" class="Clust (strict)"("Visible"=FALSE) -> ()  [unwired: 2 in, 2 out]
          }
          frame True {
            n283 = property on="About" class="Clust (strict)"("Visible"=TRUE) -> ()  [unwired: 2 in, 2 out]
          }
        }
      }
      event "Calibration": Value Change {
        n284 = event-data() -> ()  [unwired: 1 in, 6 out]
        n285 = local read "Calibration"() -> (w381:bool)
        n286 = case shown="False" w381 {
          frame False {
            n287 = property on="Calibration 2" class="TabCtl (strict)"("Visible"=FALSE) -> ()  [unwired: 2 in, 2 out]
            n288 = local write "Cal Password"("" ("Cal Password")) -> ()
          }
          frame True {
            n289 = property on="Calibration 2" class="TabCtl (strict)"("Visible"=TRUE) -> ()  [unwired: 2 in, 2 out]
            n290 = local write "Cal Password"("" ("Cal Password")) -> ()
          }
        }
        n291 = property on="Wrong Password" class="Str"("Visible"=FALSE) -> ()  [unwired: 2 in, 2 out]
      }
      event "Cal Password": Value Change {
        n292 = event-data() -> ()  [unwired: 1 in, 6 out]
        n293 = local read "Cal Password"() -> (w389:string)
        n294 = call <vilib>:"Trim Whitespace.vi"("string"=w389) -> ("trimmed string"=w388:string)  [unwired: 1 in]
        n295 = Equal?(x=w388, y="Cal@321") -> (x = y?=w386:bool)
        n296 = case shown="True" w386 {
          frame False {
            n297 = property on="Wrong Password" class="Str"("Visible"=TRUE) -> ()  [unwired: 2 in, 2 out]
          }
          frame True {
            n298 = property on="Wrong Password" class="Str"("Visible"=FALSE) -> ()  [unwired: 2 in, 2 out]
            n299 = local write "Main Tab"(T2."About" ("Main Tab")) -> ()
            n300 = local write "Cal Password"("" ("Cal Password")) -> ()
            n301 = local write "Main Dashboard Buttons"(T1."About" ("Main Dashboard Buttons")) -> ()
            n302 = local write "Tab Control 5"(T7."Temperature Calibration" ("Tab Control 5")) -> ()
            n303 = property on="Calibration 2" class="TabCtl (strict)"("Visible"=FALSE) -> ()  [unwired: 2 in, 2 out]
            n304 = property on="Tab Control 5" class="TabCtl (strict)"("Tabs Visible?"=FALSE ("Page Labels Display Visible?")) -> ()  [unwired: 2 in, 2 out]
            n305 = local write "Calibration"(FALSE ("Calibration")) -> ()
          }
        }
      }
      event "Quit": Value Change {
        n306 = event-data() -> ()  [unwired: 1 in, 6 out]
      }
    }
    n307 = Wait (ms)(milliseconds to wait=u32 100) -> ()  [unwired: 1 out]
  }
  n308 = local write "Auto stop temp"(w9) -> ()
  n309 = local write "main tab sub"(enum32{"Page 1", "Page 2"}."Page 1" ("main tab sub")) -> ()
  n310 = local write "USERNAME"(w28) -> ()
  n311 = local write "Main Tab"(T2."HOME" ("Main Tab")) -> ()
  n312 = local write "USER ID"(w28) -> ()
  n313 = property on="Auto Scar Check  2" class="Clust (strict)"("Visible"=w9) -> (error out=w13:errorcluster)  [unwired: 2 in, 1 out]
  n314 = property on="Quit" class="Bool (strict)"("Value"=FALSE ("Quit")) -> (error out=w30:errorcluster)  [unwired: 2 in, 1 out]
  n315 = while {
    shift-right: [w401] -> _
    shift-left: "Enum - Selector" -> [w402]
    stop <- w403 stop-if-true
    # "Auto Start Logic Loop"
    n316 = case shown="\"close\"" w402 {
      tunnel: [w406 w412 w423 w455 w486 Auto_Start_enum."Exit" ("Enum - Selector") Auto_Start_enum."Init" ("Enum - Selector")] -> w401
      frame "Init", Default {
        n317 = local read "Auto Start Test"() -> (w405:bool)
        n318 = Select(t=Auto_Start_enum."Humidity & Temperature On" ("Enum - Selector"), s=w405, f=Auto_Start_enum."Init") -> (s? t:f=w406:T10)
      }
      frame "Humidity & Temperature On" {
        n319 = flat-sequence {
          tunnel: [Auto_Start_enum."Reach point" ("Enum - Selector")] -> w409
          frame #0 {
            w413 = T15."Disabled and Grayed Out" ("Disabled")
            w414 = TRUE ("Heater Button")
            n320 = property on="Humidity" class="Bool (strict)"("DisabledEnum"=w413) -> ()  [unwired: 2 in, 2 out]
            n321 = property on="Heater Button" class="Bool (strict)"("DisabledEnum"=w413) -> ()  [unwired: 2 in, 2 out]
            n322 = local write "Heater Button"(w414) -> ()
            n323 = local write "Humidity"(w414) -> ()
          }
          frame #1 {
            n324 = Wait (ms)(milliseconds to wait=u32 1000) -> ()  [unwired: 1 out]
          }
          frame #2 {
            w416 = TRUE ("Reach point temp")
            n325 = local write "Reach point Humidity"(w416) -> ()
            n326 = local write "Reach point temp"(w416) -> ()
          }
        }
        n327 = local read "Auto Start Test"() -> (w411:bool)
        n328 = Not(x=w411) -> (.not. x?=w410:bool)
        n329 = Select(t=Auto_Start_enum."close", s=w410, f=w409) -> (s? t:f=w412:T10)
      }
      frame "Reach point" {
        w424 = TRUE ("PAUSE")
        w432 = 1.0 ("y")
        w435 = 1.0 ("y")
        n330 = local read "Set Temperature:"() -> (w436:dbl)
        n331 = local read "Set Humidity:"() -> (w431:dbl)
        n332 = local read "Humidity ( %RH )"() -> (w437:dbl)
        n333 = Add(x=w436, y=w435) -> (x+y=w434:dbl)
        n334 = Subtract(x=w436, y=w435) -> (x-y=w433:dbl)
        n335 = Add(x=w431, y=w432) -> (x+y=w430:dbl)
        n336 = Subtract(x=w431, y=w432) -> (x-y=w429:dbl)
        n337 = local read "TEMP"() -> (w438:dbl)
        n338 = In Range and Coerce(upper limit=w430, x=w437, lower limit=w429) -> (In Range?=w418:bool)  [unwired: 1 out]
        n339 = In Range and Coerce(upper limit=w434, x=w438, lower limit=w433) -> (In Range?=w419:bool)  [unwired: 1 out]
        n340 = case shown="True" w418 {
          frame False {
          }
          frame True {
            n341 = case shown="True" "Reach point Humidity" {
              selector: "Reach point Humidity" -> [_ w444]
              frame False {
              }
              frame True {
                n342 = local read "EVENT LOG"() -> (w441:string)
                n343 = Not(x=w444) -> (.not. x?=w443:bool)
                n344 = local write "Reach point Humidity"(w443) -> ()
                n345 = call "Event Log.vi"("Content"="Target Humidity reached", "EVENT LOG"=w441) -> ("EVENT LOG"=w442:string)  [unwired: 8 in, 1 out]
                n346 = local write "EVENT LOG"(w442) -> ()
              }
            }
          }
        }
        n347 = case shown="True" w419 {
          frame False {
          }
          frame True {
            n348 = case shown="True" "Reach point temp" {
              selector: "Reach point temp" -> [_ w450]
              frame False {
              }
              frame True {
                n349 = local read "EVENT LOG"() -> (w447:string)
                n350 = Not(x=w450) -> (.not. x?=w449:bool)
                n351 = local write "Reach point temp"(w449) -> ()
                n352 = call "Event Log.vi"("Content"="Target Temperature reached", "EVENT LOG"=w447) -> ("EVENT LOG"=w448:string)  [unwired: 8 in, 1 out]
                n353 = local write "EVENT LOG"(w448) -> ()
              }
            }
          }
        }
        n354 = local read "Auto Start Test"() -> (w422:bool)
        n355 = And(x=w419, y=w418) -> (x .and. y?=w428:bool)
        n356 = Select(t=Auto_Start_enum."Maintain Stage" ("Enum - Selector"), s=w428, f=Auto_Start_enum."Reach point" ("Enum - Selector")) -> (s? t:f=w425:T10)
        n357 = Not(x=w422) -> (.not. x?=w421:bool)
        n358 = Select(t=Auto_Start_enum."close", s=w421, f=w425) -> (s? t:f=w423:T10)
        n359 = call "ELAPSED TIMER VI.vi"("RESET"=w424, "PAUSE"=w424) -> ()  [unwired: 7 in, 3 out]
      }
      frame "Maintain Stage" {
        w464 = 2.0 ("y")
        w463 = 1.0 ("y")
        # "Humidity and  temperatures Set Point  have been reached"
        n360 = local read "Set Temperature:"() -> (w470:dbl)
        n361 = local read "Set Humidity:"() -> (w467:dbl)
        n362 = local read "Humidity ( %RH )"() -> (w471:dbl)
        n363 = Add(x=w470, y=w463) -> (x+y=w469:dbl)
        n364 = Subtract(x=w470, y=w463) -> (x-y=w468:dbl)
        n365 = local read "TEMP"() -> (w472:dbl)
        n366 = Add(x=w467, y=w464) -> (x+y=w466:dbl)
        n367 = Subtract(x=w467, y=w464) -> (x-y=w465:dbl)
        n368 = In Range and Coerce(upper limit=w469, x=w472, lower limit=w468) -> (In Range?=w462:bool)  [unwired: 1 out]
        n369 = In Range and Coerce(upper limit=w466, x=w471, lower limit=w465) -> (In Range?=w461:bool)  [unwired: 1 out]
        n370 = And(x=w462, y=w461) -> (x .and. y?=w460:bool)
        n371 = Not(x=w460) -> (.not. x?=w459:bool)
        n372 = call "ELAPSED TIMER VI.vi"("TARGET"=60.0, "RESET"=w459, "PAUSE"=FALSE) -> ("ELAPSED INDICATION"=w456:bool)  [unwired: 6 in, 2 out]
        n373 = case shown="True" w456 {
          tunnel: w456 -> [_ w475]
          tunnel: [Auto_Start_enum."Maintain Stage" ("Enum - Selector") w474] -> w454
          frame False {
          }
          frame True {
            n374 = stacked-sequence {
              tunnel: w475 -> [_ _ _ _ _]
              tunnel: [_ _ _ _ Auto_Start_enum."Start Stage" ("Enum - Selector")] -> w474
              frame #0 {
                n375 = local read "EVENT LOG"() -> (w477:string)
                n376 = call "Event Log.vi"("Content"="Humidity and temperature set point has stabilized.", "EVENT LOG"=w477) -> ("EVENT LOG"=w478:string)  [unwired: 8 in, 1 out]
                n377 = local write "EVENT LOG"(w478) -> ()
              }
              frame #1 {
                n378 = Wait (ms)(milliseconds to wait=u32 100) -> ()  [unwired: 1 out]
              }
              frame #2 {
                n379 = local read "EVENT LOG"() -> (w481:string)
                n380 = call "Event Log.vi"("Content"="Auto Test Started", "EVENT LOG"=w481) -> ("EVENT LOG"=w482:string)  [unwired: 8 in, 1 out]
                n381 = local write "EVENT LOG"(w482) -> ()
              }
              frame #3 {
                w483 = TRUE ("RUN")
                n382 = local write "RUN"(w483) -> ()
                "Auto Start Temp" <- w483
              }
              frame #4 {
              }
            }
          }
        }
        n383 = local read "Auto Start Test"() -> (w453:bool)
        n384 = Not(x=w453) -> (.not. x?=w452:bool)
        n385 = Select(t=Auto_Start_enum."close", s=w452, f=w454) -> (s? t:f=w455:T10)
      }
      frame "Start Stage" {
        w485 = TRUE ("PAUSE")
        n386 = local read "Auto Start Test"() -> (w490:bool)
        n387 = Not(x=w490) -> (.not. x?=w489:bool)
        n388 = Select(t=Auto_Start_enum."close" ("Enum - Selector"), s=w489, f=Auto_Start_enum."Start Stage" ("Enum - Selector")) -> (s? t:f=w486:T10)
        n389 = call "ELAPSED TIMER VI.vi"("RESET"=w485, "PAUSE"=w485) -> ()  [unwired: 7 in, 3 out]
      }
      frame "close" {
        w491 = FALSE ("Heater Button")
        n390 = local write "RUN"(w491) -> ()
        n391 = local write "Heater Button"(w491) -> ()
        n392 = local write "Humidity"(w491) -> ()
        n393 = local write "Auto Start Test"(w491) -> ()
      }
      frame "Exit" {
      }
    }
    n394 = Wait (ms)(milliseconds to wait=u32 100) -> ()  [unwired: 1 out]
    n395 = local read "Quit"() -> (w403:bool)
  }
  n396 = while {
    stop <- w520 stop-if-true
    w503 = errorcluster {"status"=FALSE, "code"=0, "source"=""} ("error in (no error) 3")
    # "this loop is for manual report generation"
    n397 = local read "Confirm Measrurement"() -> (w502:bool)
    n398 = case shown="True" w502 {
      selector: w502 -> [_ w610]
      tunnel: errorcluster {"status"=FALSE, "code"=0, "source"=""} ("error in (no error) 3") -> [_ w611]
      tunnel: [_ w609] -> _
      frame False {
      }
      frame True {
        n399 = stacked-sequence {
          tunnel: w611 -> [_ w644 _]
          tunnel: w610 -> [_ _ w751]
          tunnel: [_ w632 _] -> w609
          frame #0 {
            n400 = String To Path(string="C:\\LAB-IQ\\Image Calibrate v01.dcf") -> (path=w614:path)
            n401 = Open/Create/Replace File ("Open File")(file path (use dialog)=w614) -> (refnum out=w615:refnum<file>)  [unwired: 5 in, 2 out]
            n402 = for {
              N: 4 -> [_]
              tunnel: w615 -> [w621]
              i -> [w617]
              n403 = Read from Text File ("Read File")(file (use dialog)=w621) -> (text=w622:string)  [unwired: 3 in, 3 out]
              n404 = String Subset(string=w622, offset (0)=6, length (rest)=10 ("length (rest)")) -> (substring=w618:string)
              n405 = Fract/Exp String To Number(string=w618) -> (number=w616:dbl)  [unwired: 3 in, 1 out]
              n406 = case shown="3" w617 {
                tunnel: w616 -> [w623 w624 _ w625 _]
                frame 0 {
                  n407 = local write "5x Gain"(w623) -> ()
                }
                frame 1 {
                  n408 = local write "10x Gain"(w624) -> ()
                }
                frame 2 {
                }
                frame 3 {
                  n409 = local write "100x gain"(w625) -> ()
                }
                frame 4, Default {
                }
              }
            }
          }
          frame #1 {
            n410 = local read "TEST STANDARD"() -> (w627:T3)
            n411 = case shown="\"ISO 12156\"" w627 {
              tunnel: ["ASTM D6079" "ISO 12156"] -> w626
              frame "ASTM D6079", Default {
              }
              frame "ISO 12156" {
              }
            }
            n412 = call "IMAGE ANALYSIS.vi"("Enum"=POST_ANALYSIS_ENUM."GET MEASUREMENTS", "error in"=w644) -> ("error out"=w651:errorcluster)  [unwired: 8 in, 1 out]
            n413 = local read "Magnification :"() -> (w637:string)
            n414 = call "Stall Data Flow.vim"("value in"=w651, "milliseconds to wait"=u32 1000) -> ("value out"=w650:errorcluster)  [unwired: 1 out]
            n415 = local read "Test File List :"() -> (w648:string)
            n416 = case shown="\"10x\"" w637 {
              tunnel: [w687 w688] -> w635
              frame "5x", Default {
                n417 = local read "5x Gain"() -> (w687:dbl)
              }
              frame "10x" {
                # "5x"
                n418 = local read "10x Gain"() -> (w688:dbl)
              }
            }
            n419 = call "IMAGE ANALYSIS.vi"("Enum"=POST_ANALYSIS_ENUM."READ", "error in"=w650) -> ("error out"=w647:errorcluster, "data out"=w638:string)  [unwired: 8 in]
            n420 = Match Pattern(string=w638, regular expression="\"type\": ") -> (after substring=w642:string)  [unwired: 1 in, 3 out]
            n421 = call "IMAGE PATH CREATION PY.vi"("error in (no error)"=w647, "File Name :"=w648) -> ("error out"=w646:errorcluster, "File Path"=w634:path, "File Path String:"=w629:string)  [unwired: 7 in]
            n422 = Match Pattern(string=w642, regular expression=",") -> (before substring=w628:string)  [unwired: 1 in, 3 out]
            n423 = local read "Calibration Tab"() -> (w631:enum32{"Measrument", "Calibrate"})
            n424 = call "Stall Data Flow.vim"("value in"=w646, "milliseconds to wait"=u32 250) -> ("value out"=w630:errorcluster)  [unwired: 1 out]
            n425 = Equal?(x=w628, y="\"rectangle\"") -> (x = y?=w639:bool)
            n426 = case shown="False" w639 {
              tunnel: w638 -> [w693 w748]
              tunnel: w635 -> [_ w739]
              tunnel: cluster{"major":dbl, "minor":dbl, "average":dbl} {"major"=0.0, "minor"=0.0, "average"=0.0} -> [w691 w735]
              tunnel: [w690 w732] -> w633
              tunnel: w628 -> [w692 _]
